vi "CleanedSubversionRevision.vi"(11 "File Path Control":path caption="File Path Control (leave blank to use Constants_Global value of EnFlo SW Folder)") -> (1 "Revision":u32, 2 "CleanRevisionString":string)   [LabVIEW 2017]
uses:
  Globals/Constants_global.vi
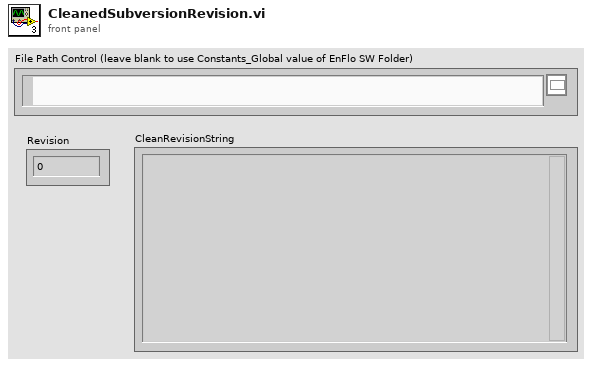
[diagram p1: front panel]
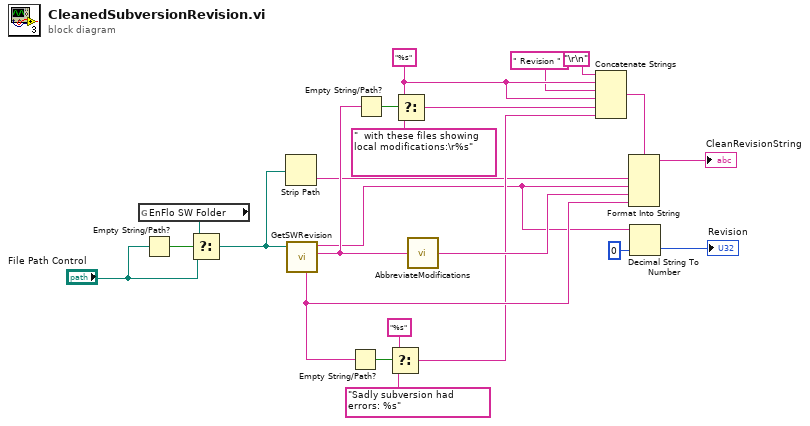
[diagram p0: block diagram]
diagram:
  w3 = "%s" ("format string")
  n1 = global read "Constants_global.vi" "EnFlo SW Folder"() -> (w8:path)
  n2 = Empty String/Path?(string/path="File Path Control") -> (empty?=w9:bool)
  n3 = Select(t=w8, s=w9, f="File Path Control") -> (s? t:f=w6:path)
  n4 = Strip Path(path=w6) -> (name=w4:string)  [unwired: 1 out]
  n5 = call "GetSWRevision.vi"("File Path Control"=w6) -> ("LocalModifications"=w21:string, "OverallRevision"=w5:string, "standard error"=w20:string)  [unwired: 5 in, 3 out]
  n6 = Empty String/Path?(string/path=w20) -> (empty?=w17:bool)
  n7 = Empty String/Path?(string/path=w21) -> (empty?=w12:bool)
  n8 = Select(t="%s" ("format string"), s=w17, f="Sadly subversion had errors: %s" ("format string")) -> (s? t:f=w19:string)
  n9 = Select(t=w3, s=w12, f="  with these files showing local modifications:\r%s" ("format string")) -> (s? t:f=w14:string)
  n10 = call "AbbreviateModifications.vi"("svnString"=w21) -> ("VInames"=w22:string)  [unwired: 4 in]
  n11 = Concatenate Strings("\r\n", w3, " Revision " ("string"), w3, w14, w19) -> (w15:string)
  n12 = Format Into String(format string=w15, w4, w5, w22, w20) -> (resulting string=→"CleanRevisionString":string)  [unwired: 2 in, 1 out]
  n13 = Decimal String To Number(string=w5, default (0L)=u32 0 ("default (0 I32)")) -> (number=→"Revision":u32)  [unwired: 1 in, 1 out]
